vi "Manual_Control_Main.vi"() -> ()   [LabVIEW 2024]
uses:
  <vilib>/Platform/TimedLoop/XDataNode/timing_clust.ctl
  <vilib>/Platform/TimedLoop/XDataNode/nitl_modes.ctl
  <vilib>/Platform/TimedLoop/XDataNode/wakeup.ctl
  <vilib>/addons/Maxon Motor/EPOS2 CANopen/CANopen/sbCANopenBaseClass.lvclass
  <vilib>/platform/TimedLoop/XDataNode/XDataNode.xnode
  <vilib>/Platform/TimedLoop/XDataNode/XDNodeRunTimeDep.lvlib
panel:
  out "ResetPID":bool
  in  "Motor_index":i32[](array[numeric])=[3, 6, 9, 12, 2, 7, 8, 13, 4, 5, 10, 11, 1, 14]
  out "canERROR":errorcluster[][](array[cluster])
  in  "Control Mode":string="O"
  in  "goal_Tensions":dbl[](array[numeric])=[0.0, 0.0, 0.0, 0.0, 0.0, 0.0, 0.0, 0.0, 0.0, 0.0, 0.0, 0.0, 0.0, 0.0]
  in  "TARE":bool
  in  "curr_Tensions":dbl[](array[numeric])
  out "DAQ Error":errorcluster
  out "Write Late?":bool
  out "Write Time [us]":i64
  in  "Tare_Tensions":dbl[](array[numeric])=[1.6875269817998764, 0.7228096971601798, 1.962272927280566, 2.6696462364433735, 2.7003690389898463, 3.088938448864716, 1.6430905755314908, 3.0754139877790347, 3.5546581214666455, 3.2737863413382597, 4.727265898547672, 2.6001067118162604, 1.980007529135911, 1.8614502099489874]
  in  "STOP CONTROLLER":bool
  # "2\n\n3\n\n4\n\n5\n\n6\n\n7\n\n8\n\n9\n\n10\n\n11\n\n12\n\n13"
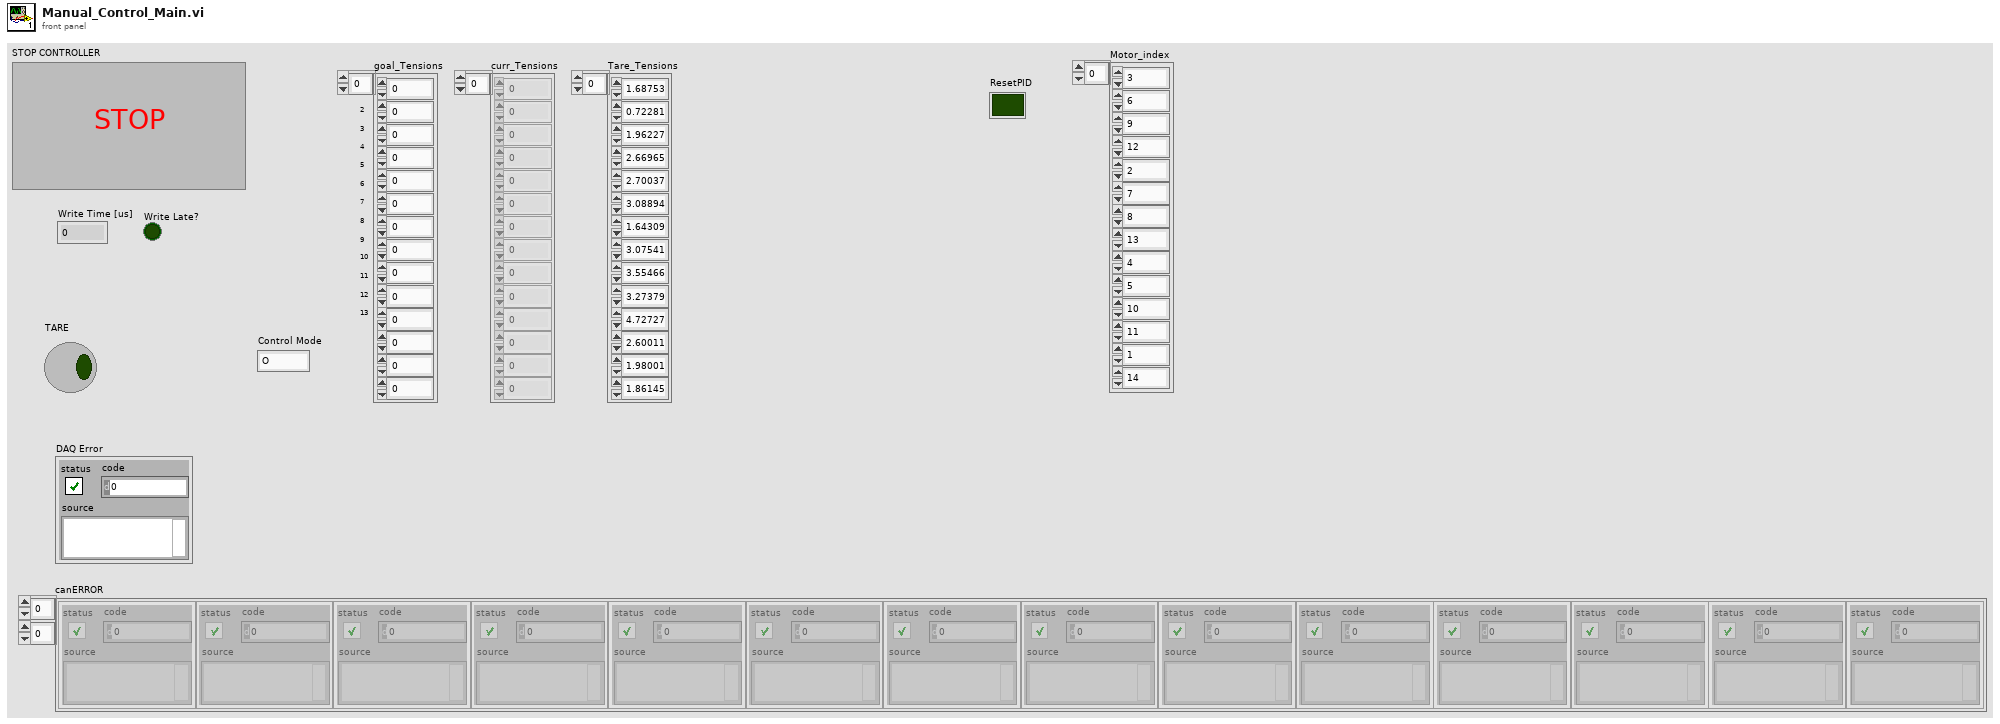
[diagram p1: front panel]
types:
  T1 = typedef "XDNodeRunTimeDep.lvlib/timing_clust.ctl" = cluster{"Expected End [f-1]":u64, "Actual End [f-1]":u64, "Finished Late? [f-1]":bool, "Expected End [i-1]":u64, "Actual End [i-1]":u64, "Finished Late? [i-1]":bool, "Expected Start [i]":u64, "Actual Start [i]":u64, "Expected Start [f]":u64, "Actual Start [f]":u64, "Source Name":string, "Structure Name":string, "Period":i64, "Deadline":i64, "Offset":i64, "Start":i64, "Priority":i32, "Timeout":i32, "Mode":T2, "Wakeup Reason":T3, "Error":errorcluster, "Source Type":string, "Secondary Source Type":string, "Global End Time":u64, "Global Start Time":u64, "Frame Duration":u64, "Iteration Duration":u64, "Assigned CPU":i32, "I/O Scan Engine Mode":u32}
  T2 = typedef "XDNodeRunTimeDep.lvlib/nitl_modes.ctl" = enum32{"No Change", "Process missed periods, maintain original phase", "Discard missed periods, maintain original phase", "Process missed periods, ignore original phase", "Discard missed periods, ignore original phase"}
  T3 = typedef "XDNodeRunTimeDep.lvlib/wakeup.ctl" = enum32{"Normal", "Aborted", "Asynchronous wakeup", "Timing source error", "Timed loop error", "Timeout"}
  T4 = cluster{"curr_Tensions":dbl[], "goal_Tensions":dbl[]}
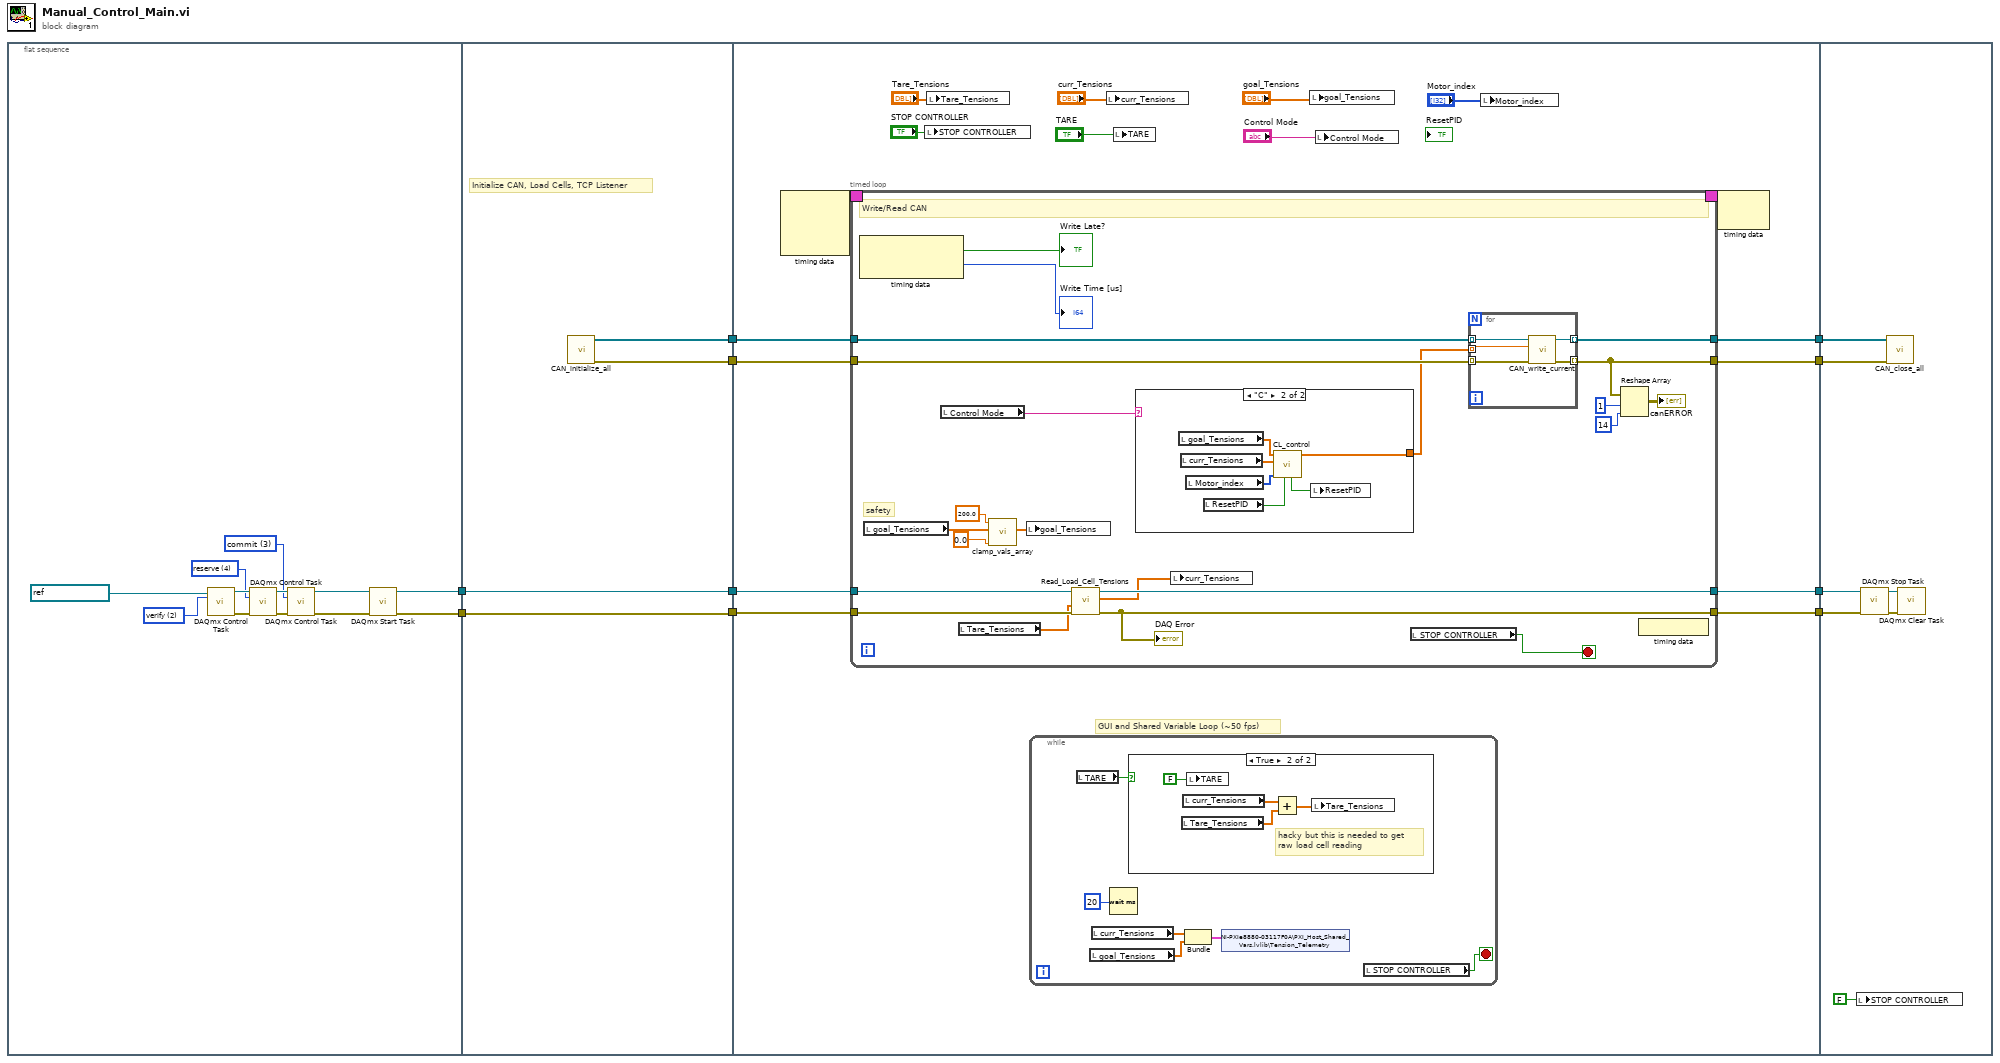
[diagram p0: block diagram]
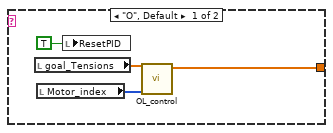
[diagram p3: hidden frame]
diagram:
  n1 = flat-sequence {
    tunnel: [w12] -> w2
    tunnel: [w11] -> w1
    tunnel: [w25] -> w10
    tunnel: [w26] -> w9
    tunnel: [w24] -> w6
    tunnel: [w23] -> w5
    tunnel: w2 -> [w24]
    tunnel: w1 -> [w23]
    tunnel: w10 -> [w41]
    tunnel: w9 -> [w40]
    tunnel: [w39] -> w8
    tunnel: [w38] -> w7
    tunnel: w6 -> [w36]
    tunnel: w5 -> [w35]
    tunnel: [w34] -> w4
    tunnel: [w33] -> w3
    tunnel: w8 -> [w103]
    tunnel: w7 -> [w102]
    tunnel: w4 -> [w99]
    tunnel: w3 -> [w98]
    frame #0 {
      w16 = 3 items=["verify"=2, "reserve"=4, "commit"=3, "unreserve"=5, "abort"=6] ("action")
      w15 = 4 items=["verify"=2, "reserve"=4, "commit"=3, "unreserve"=5, "abort"=6] ("action")
      w13 = 2 items=["verify"=2, "reserve"=4, "commit"=3, "unreserve"=5, "abort"=6] ("action")
      n2 = call <vilib>:"DAQmx Control Task.vi"("task/channels in"=refnum<k21> "SCI_TenSen", "action"=w13) -> ("task out"=w17:refnum<k21>, "error out"=w19:errorcluster)  [unwired: 12 in]
      n3 = call <vilib>:"DAQmx Control Task.vi"("task/channels in"=w17, "action"=w15, "error in"=w19) -> ("task out"=w18:refnum<k21>, "error out"=w20:errorcluster)  [unwired: 11 in]
      n4 = call <vilib>:"DAQmx Control Task.vi"("task/channels in"=w18, "action"=w16, "error in"=w20) -> ("task out"=w21:refnum<k21>, "error out"=w22:errorcluster)  [unwired: 11 in]
      n5 = call <vilib>:"DAQmx Start Task.vi"("task/channels in"=w21, "error in"=w22) -> ("task out"=w12:refnum<k21>, "error out"=w11:errorcluster)  [unwired: 12 in]
    }
    frame #1 {
      # "Initialize CAN, Load Cells, TCP Listener"
      n6 = call "CAN_initialize_all.vi"() -> ("Array of Canopen Sessions"=w26:refnum<class "sbCANopenBaseClass.lvclass">[], "Array of Error out's"=w25:errorcluster[])  [unwired: 5 in]
    }
    frame #2 {
      # "GUI and Shared Variable Loop (~50 fps)"
      n7 = node-c288() -> (w43:T1)  [unwired: 3 in]
      n8 = timed-loop {
        tunnel: w41 -> [w67]
        tunnel: [w59] -> w39
        timing: w43 -> [_]
        timing-out: [_] -> w42
        tunnel: w40 -> [w68]
        tunnel: [w72] -> w38
        tunnel: w36 -> [w71]
        tunnel: w35 -> [w70]
        tunnel: [w69] -> w34
        tunnel: [w66] -> w33
        stop <- w73 stop-if-true
        # "safety"
        # "Write/Read CAN"
        n9 = node-c288() -> (→"Write Late?":bool, →"Write Time [us]":i64)  [unwired: 1 in]
        n10 = local read "goal_Tensions"() -> (w54:dbl[])
        n11 = local read "Control Mode"() -> (w64:string)
        n12 = local read "Tare_Tensions"() -> (w65:dbl[])
        n13 = call "clamp_vals_array.vi"("Min Val"=0.0, "Input Array"=w54, "Max Val"=200.0) -> ("Output Array"=w55:dbl[])  [unwired: 8 in]
        n14 = local write "goal_Tensions"(w55) -> ()
        n15 = call "Read_Load_Cell_Tensions.vi"("error in (no error)"=w70, "Tare Tension"=w65, "Refnum in"=w71) -> ("error out"=w66:errorcluster, "Measured Cable Tensions"=w63:dbl[], "Refnum out"=w69:refnum<k21>)  [unwired: 4 in]
        "DAQ Error" <- w66
        n16 = case shown="\"C\"" w64 {
          tunnel: [w79 w85] -> w62
          frame "O", Default {
            n17 = local read "goal_Tensions"() -> (w76:dbl[])
            n18 = local read "Motor_index"() -> (w78:i32[])
            n19 = local write "ResetPID"(TRUE) -> ()
            n20 = call "OL_control.vi"("Motor_index"=w78, "goal_Tensions"=w76) -> ("can_Current"=w79:dbl[])  [unwired: 9 in]
          }
          frame "C" {
            n21 = local read "goal_Tensions"() -> (w80:dbl[])
            n22 = local read "curr_Tensions"() -> (w81:dbl[])
            n23 = local read "Motor_index"() -> (w84:i32[])
            n24 = local read "ResetPID"() -> (w83:bool)
            n25 = call "CL_control.vi"("ResetPID"=w83, "Motor_index"=w84, "curr_Tensions"=w81, "goal_Tensions"=w80) -> ("can_Current"=w85:dbl[], "Reset PID (output)"=w82:bool)  [unwired: 6 in]
            n26 = local write "ResetPID"(w82) -> ()
          }
        }
        n27 = local write "curr_Tensions"(w63) -> ()
        n28 = local read "STOP CONTROLLER"() -> (w73:bool)
        n29 = for {
          tunnel: [w87] -> w72 mode=indexing
          tunnel: [w88] -> w59 mode=indexing
          tunnel: w68 -> [w90] mode=indexing
          tunnel: w67 -> [w89] mode=indexing
          tunnel: w62 -> [w86] mode=indexing
          n30 = call "CAN_write_current.vi"("error in"=w89, "Current Command [mA]"=w86, "CANopen Session In"=w90) -> ("error out"=w88:errorcluster, "CANopen Session Out"=w87:refnum<class "sbCANopenBaseClass.lvclass">)  [unwired: 7 in]
        }
        n31 = Reshape Array(w59, 1 ("dimension size"), 14 ("dimension size")) -> (→"canERROR":errorcluster[][])
        n32 = node-c288() -> ()  [unwired: 1 out]
      }
      n33 = local write "STOP CONTROLLER"("STOP CONTROLLER") -> ()
      n34 = local write "Tare_Tensions"("Tare_Tensions") -> ()
      n35 = while {
        stop <- w49 stop-if-true
        n36 = local read "TARE"() -> (w48:bool)
        n37 = local read "goal_Tensions"() -> (w44:dbl[])
        n38 = local read "curr_Tensions"() -> (w47:dbl[])
        n39 = Wait (ms)(milliseconds to wait=u32 20) -> ()  [unwired: 1 out]
        n40 = case shown="True" w48 {
          frame False {
          }
          frame True {
            # "hacky but this is needed to get \nraw load cell reading"
            n41 = local read "Tare_Tensions"() -> (w51:dbl[])
            n42 = local read "curr_Tensions"() -> (w52:dbl[])
            n43 = local write "TARE"(FALSE ("TARE")) -> ()
            n44 = Add(x=w52, y=w51) -> (x+y=w53:dbl[])
            n45 = local write "Tare_Tensions"(w53) -> ()
          }
        }
        n46 = Bundle("curr_Tensions"=w47, "goal_Tensions"=w44) -> (w46:T4)  [unwired: 1 in]
        n47 = shared-variable "NI-PXIe8880-03117F0A\\PXI_Host_Shared_Vars.lvlib\\Tension_Telemetry"(w46) -> ()  [unwired: 1 in, 1 out]
        n48 = local read "STOP CONTROLLER"() -> (w49:bool)
      }
      n49 = local write "curr_Tensions"("curr_Tensions") -> ()
      n50 = local write "TARE"("TARE") -> ()
      n51 = local write "goal_Tensions"("goal_Tensions") -> ()
      n52 = local write "Control Mode"("Control Mode") -> ()
      n53 = local write "Motor_index"("Motor_index") -> ()
      n54 = node-c288(w42) -> ()  [unwired: 1 out]
    }
    frame #3 {
      n55 = local write "STOP CONTROLLER"(FALSE ("STOP CONTROLLER")) -> ()
      n56 = call <vilib>:"DAQmx Stop Task.vi"("task/channels in"=w99, "error in"=w98) -> ("task out"=w100:refnum<k21>, "error out"=w101:errorcluster)  [unwired: 12 in]
      n57 = call "CAN_close_all.vi"("Input Error out array"=w103, "Input CANopen Sessions array"=w102) -> ()  [unwired: 10 in]
      n58 = call <vilib>:"DAQmx Clear Task.vi"("task in"=w100, "error in"=w101) -> ()  [unwired: 13 in, 1 out]
    }
  }
